vi "Shift_Value_CH0_calibration_Rev03x.vi"(0 "IN1 Shift Val1":dbl, 1 "Enable memory wright":bool, 3 "Range IN1":dbl, 4 "USB Interface Name":refnum<visa-resource-name>="COM3", 5 "Input buffer size":u32=16384, 7 "error in (no error)":errorcluster, 13 "WRITE":bool, 27 "Sign Value":dbl) -> (8 "MB address":string, 9 "MB value":u8 format="%x", 10 "Reply 1":string, 12 "UB address":string, 14 "HB address":string, 15 "error out":errorcluster, 16 "LB address":string, 17 "UB value":u8 format="%x", 18 "Reply 2":string, 19 "Data string CH0":string, 20 "IN1 shift uV":dbl, 21 "IN1 shift  HEX uV":u32 format="%x", 22 "Reply 3":string, 23 "Sign Addrss":string, 24 "HB value":u8 format="%x", 25 "LB value":u8 format="%x", 26 "Reply 4":string)   [LabVIEW 2012]
panel:
  out "LB value":string
  out "HB value":string
  out "UB value":string
  out "MB value":string
  # "1. Computes address based on the input range \"Range IN\"\n2. Take absolute values of positive and negative voltage reads in uV compares them and subtracts smaller value from the larger one. The result is devided by 2.\nIf VAL1>VAL2: ( |VAL1| - |VAL2| )/ 2"
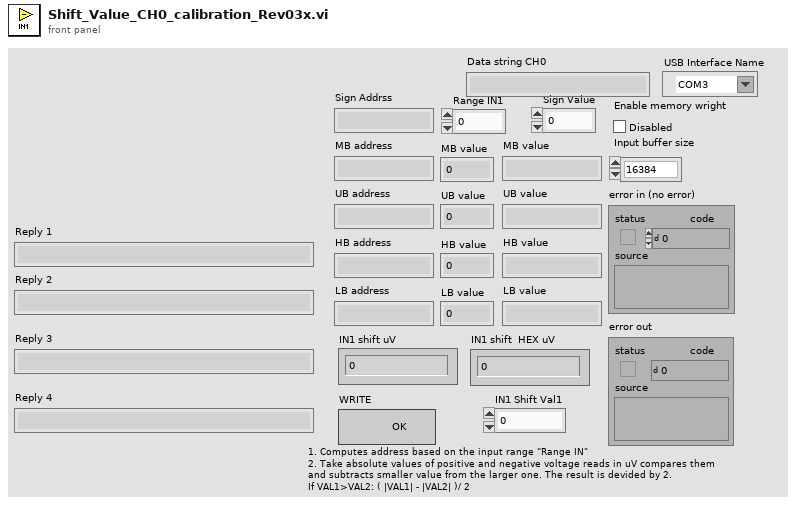
[diagram p1: front panel]
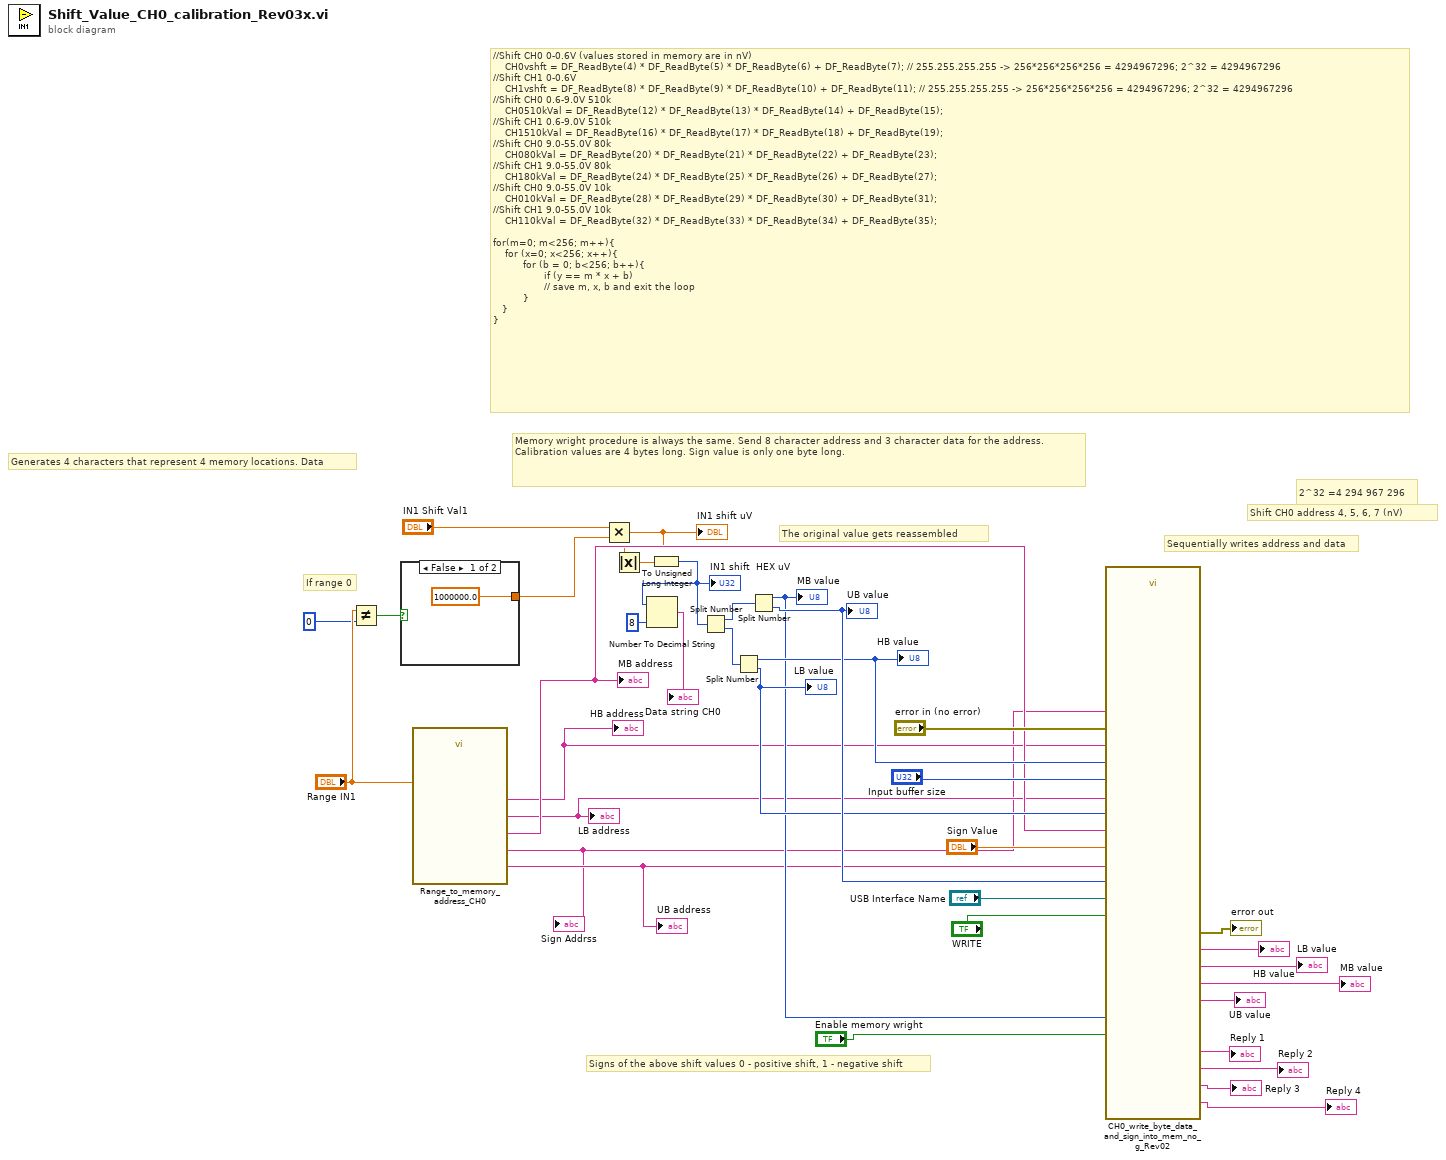
[diagram p0: block diagram]
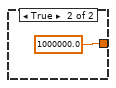
[diagram p2: hidden frame]
diagram:
  # "If range 0"
  # "Shift CH0 address 4, 5, 6, 7 (nV)"
  # "Signs of the above shift values 0 - positive shift, 1 - negative shift"
  # "The original value gets reassembled"
  # "//Shift CH0 0-0.6V (values stored in memory are in nV)     \n    CH0vshft = DF_ReadByte(4) * DF_ReadByte(5) * DF_ReadByte(6) + DF_ReadByte(7); // 255.255.255.255 -> 256*256*256*256 = 4294967296; 2^32 = 4294967296\n//Shift CH1 0-0.6V\n    CH1vshft = DF_ReadByte(8) * DF_ReadByte(9) * DF_ReadByte(10) + DF_ReadByte(11); // 255.255.255.255 -> 256*256*256*256 = 4294967296; 2^32 = 4294967296\n//Shift CH0 0.6-9.0V 510k\n    CH0510kVal = DF_ReadByte(12) * DF_ReadByte(13) * DF_ReadByte(14) + DF_ReadByte(15);\n//Shift CH1 0.6-9.0V 510k\n    CH1510kVal = DF_ReadByte(16) * DF_ReadByte(17) * DF_ReadByte(18) + DF_ReadByte(19);\n//Shift CH0 9.0-55.0V 80k            \n    CH080kVal = DF_ReadByte(20) * DF_ReadByte(21) * DF_ReadByte(22) + DF_ReadByte(23);\n//Shift CH1 9.0-55.0V 80k\n    CH180kVal = DF_ReadByte(24) * DF_ReadByte(25) * DF_ReadByte(26) + DF_ReadByte(27);\n//Shift CH0 9.0-55.0V 10k\n    CH010kVal = DF_ReadByte(28) * DF_ReadByte(29) * DF_ReadByte(30) + DF_ReadByte(31);\n//Shift CH1 9.0-55.0V 10k\n    CH110kVal = DF_ReadByte(32) * DF_ReadByte(33) * DF_ReadByte(34) + DF_ReadByte(35);\n\nfor(m=0; m<256; m++){\n    for (x=0; x<256; x++){\n          for (b = 0; b<256; b++){\n                 if (y == m * x + b)\n                 // save m, x, b and exit the loop\n          }\n   }\n}"
  # "Sequentially writes address and data"
  # "Memory wright procedure is always the same. Send 8 character address and 3 character data for the address.\nCalibration values are 4 bytes long. Sign value is only one byte long."
  # "2^32 =4 294 967 296"
  # "Generates 4 characters that represent 4 memory locations. Data"
  n1 = Not Equal?(x="Range IN1", y=0) -> (x != y?=w3:bool)
  n2 = case shown="False" w3 {
    tunnel: [1000000.0 1000000.0] -> w36
    frame False {
    }
    frame True {
    }
  }
  n3 = call "Range_to_memory_address_CH0.vi"("Range IN1"="Range IN1") -> ("LB address"=w11:string, "HB address"=w12:string, "UB address"=w13:string, "MB address"=w14:string, "Sign Addrss"=w10:string)  [unwired: 6 in]
  "MB address" <- w14
  "UB address" <- w13
  "HB address" <- w12
  "LB address" <- w11
  "Sign Addrss" <- w10
  n4 = Multiply(x="IN1 Shift Val1", y=w36) -> (x*y=w4:dbl)
  "IN1 shift uV" <- w4
  n5 = Absolute Value(x=w4) -> (abs(x)=w5:dbl)
  n6 = To Unsigned Long Integer(number=w5) -> (unsigned 32bit integer=w17:u32)
  "IN1 shift  HEX uV" <- w17
  n7 = Number To Decimal String(number=w17, width (-)=8) -> (decimal integer string=→"Data string CH0":string)
  n8 = Split Number(x=w17) -> (hi(x)=w35:u16, lo(x)=w34:u16)
  n9 = Split Number(x=w34) -> (hi(x)=w29:u8, lo(x)=w28:u8)
  "HB value" <- w29
  "LB value" <- w28
  n10 = Split Number(x=w35) -> (hi(x)=w19:u8, lo(x)=w30:u8)
  "MB value" <- w19
  "UB value" <- w30
  n11 = call "CH0_write_byte_data_and_sign_into_mem_no_g_Rev02.vi"("MB data"=w19, "UB data"=w30, "Sign addrss 8 byte"=w10, "USB Interface Name"="USB Interface Name", "HB data"=w29, "LB data"=w28, "MB addrss 8 byte"=w14, "HB addrss 8 byte"=w12, "LB addrss 8 byte"=w11, "Sign data 3 byte"="Sign Value", "WRITE DATA"="WRITE", "Input buffer size"="Input buffer size", "UB addrss 8 byte"=w13, "error in (no error)"="error in (no error)", "Enable memory wright"="Enable memory wright") -> ("Reply 1"=→"Reply 1":string, "Reply 2"=→"Reply 2":string, "MB data 3 byte"=→"MB value":string, "UB data 3 byte"=→"UB value":string, "Reply 3"=→"Reply 3":string, "error out"=→"error out":errorcluster, "HB data 3 byte"=→"HB value":string, "Reply 4"=→"Reply 4":string, "LB data 3 byte"=→"LB value":string)  [unwired: 4 in]
